vi "compare maps.vi"(10 "poolarimeter map path":path=path "test.tdms" caption="Filename", 11 "germanium map path":path=path "test.tdms" caption="Filename") -> (3 "germainium to polarimeter map":dbl[][](array[numeric]))   [LabVIEW 2018]
panel:
  out "map of germainium to polarimeter output along RF input unitary":T1(graph)
  out "Polarimeter Response Curve":cluster{dbl[], dbl[]}(graph)
  out "y offset 2":dbl
  out "y range 2":dbl
  out "x range 2":dbl
  out "x offset 2":dbl
  out "Germanium Response Curve":cluster{dbl[], dbl[]}(graph)
  out "y offset":dbl
  out "y range":dbl
  out "x range":dbl
  out "x offset":dbl
  out "Response Comparision":cluster{dbl[], dbl[]}[](graph)
  out "map of germainium to polarimeter output along RF input":T1(graph)
  out "germainium to polarimeter map unitary":dbl[][](array[numeric])
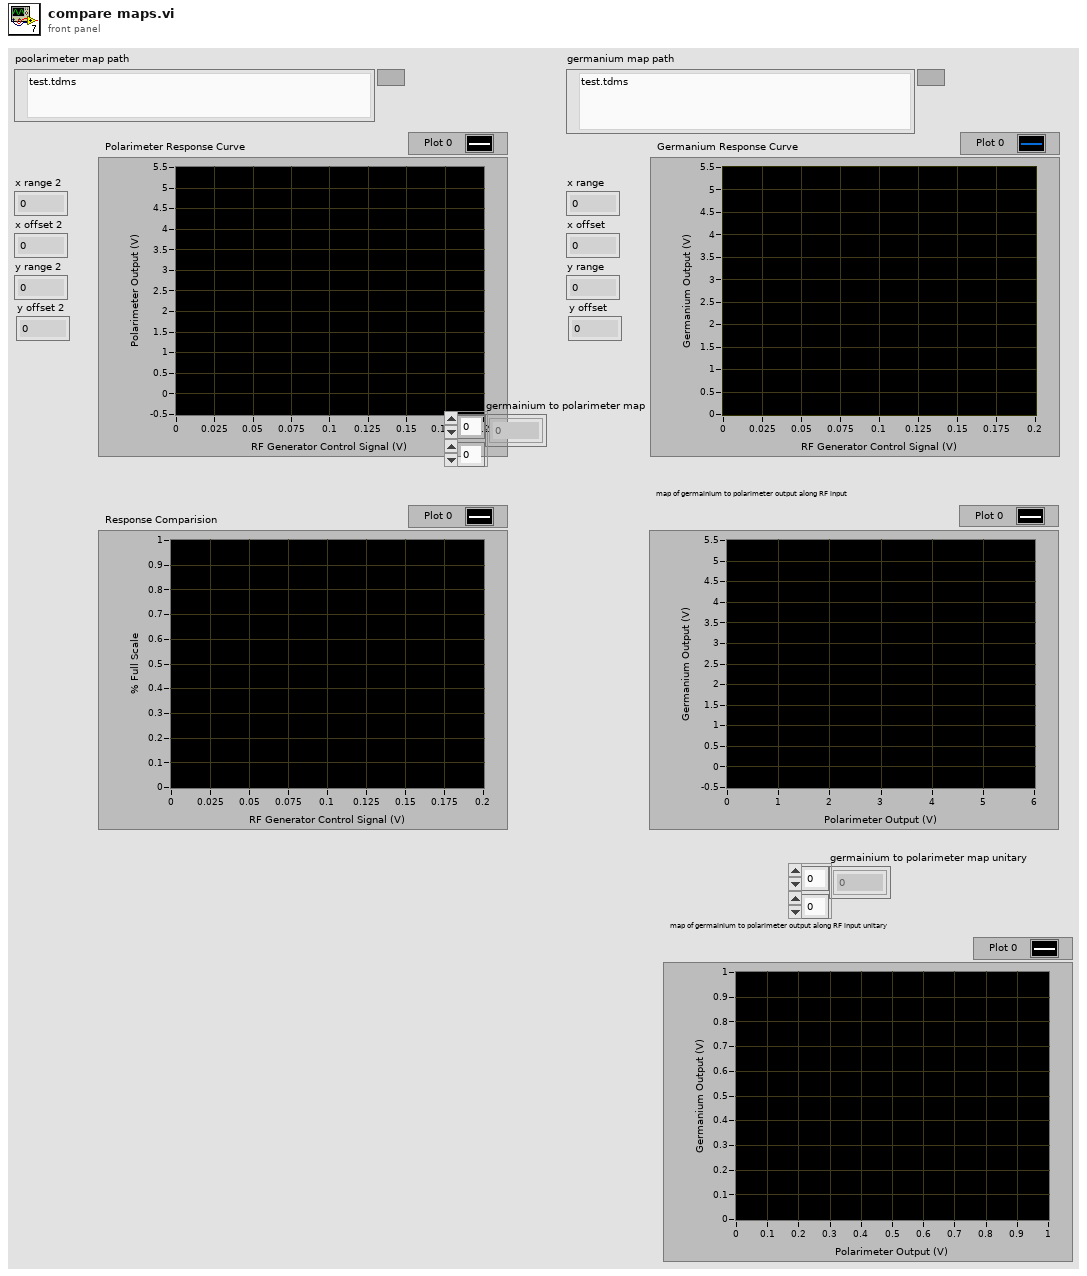
[diagram p1: front panel]
types:
  T1 = cluster{"Scaled Array":dbl[], "Scaled Array":dbl[]}
  T2 = cluster{"1N array":dbl[], "Scaled Array":dbl[]}[]
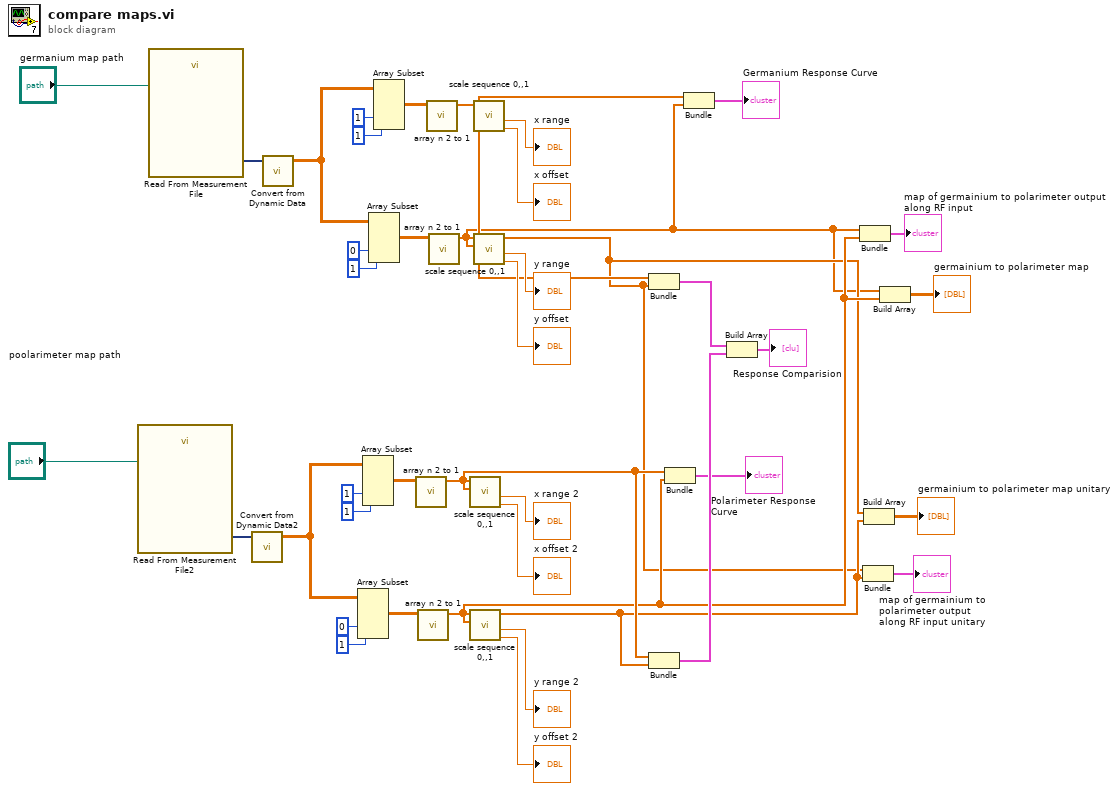
[diagram p0: block diagram]
diagram:
  n1 = call "Read From Measurement File2"("Filename"="poolarimeter map path") -> ("Signals"=w33:dynamicdata)  [unwired: 5 in, 5 out]
  n2 = call "Read From Measurement File"("Filename"="germanium map path") -> ("Signals"=w41:dynamicdata)  [unwired: 5 in, 5 out]
  n3 = call "Convert from Dynamic Data2"("Dynamic Data Type"=w33) -> ("Array"=w28:dbl[][])  [unwired: 3 in]
  n4 = call "Convert from Dynamic Data"("Dynamic Data Type"=w41) -> ("Array"=w36:dbl[][])  [unwired: 3 in]
  n5 = Array Subset(array=w28, index (col)=0 ("index"), length (col)=1 ("length")) -> (w26:dbl[][])  [unwired: 2 in]
  n6 = Array Subset(array=w28, index (col)=1 ("index"), length (col)=1 ("length")) -> (w27:dbl[][])  [unwired: 2 in]
  n7 = Array Subset(array=w36, index (col)=0 ("index"), length (col)=1 ("length")) -> (w34:dbl[][])  [unwired: 2 in]
  n8 = Array Subset(array=w36, index (col)=1 ("index"), length (col)=1 ("length")) -> (w35:dbl[][])  [unwired: 2 in]
  n9 = call "array n 2 to 1.vi"("2N array"=w27) -> ("1N array"=w8:dbl[])  [unwired: 10 in]
  n10 = call "array n 2 to 1.vi"("2N array"=w26) -> ("1N array"=w5:dbl[])  [unwired: 10 in]
  n11 = call "array n 2 to 1.vi"("2N array"=w35) -> ("1N array"=w10:dbl[])  [unwired: 10 in]
  n12 = call "array n 2 to 1.vi"("2N array"=w34) -> ("1N array"=w3:dbl[])  [unwired: 10 in]
  n13 = call "scale sequence 0,,1.vi"("Data"=w8, "map sequence"=w8) -> ("offset"=→"x offset 2":dbl, "range"=→"x range 2":dbl)  [unwired: 7 in, 1 out]
  n14 = call "scale sequence 0,,1.vi"("Data"=w5, "map sequence"=w5) -> ("offset"=→"y offset 2":dbl, "range"=→"y range 2":dbl, "Scaled Array"=w7:dbl[])  [unwired: 7 in]
  n15 = call "scale sequence 0,,1.vi"("Data"=w10, "map sequence"=w10) -> ("offset"=→"x offset":dbl, "range"=→"x range":dbl)  [unwired: 7 in, 1 out]
  n16 = call "scale sequence 0,,1.vi"("Data"=w3, "map sequence"=w3) -> ("offset"=→"y offset":dbl, "range"=→"y range":dbl, "Scaled Array"=w4:dbl[])  [unwired: 7 in]
  n17 = Bundle("1N array"=w10, "Scaled Array"=w4) -> (w22:cluster{"1N array":dbl[], "Scaled Array":dbl[]})  [unwired: 1 in]
  n18 = Bundle("1N array"=w8, "Scaled Array"=w7) -> (w16:cluster{"1N array":dbl[], "Scaled Array":dbl[]})  [unwired: 1 in]
  n19 = Bundle("1N array"=w8, "1N array"=w5) -> (→"Polarimeter Response Curve":cluster{"1N array":dbl[], "1N array":dbl[]})  [unwired: 1 in]
  n20 = Bundle("1N array"=w10, "1N array"=w3) -> (→"Germanium Response Curve":cluster{"1N array":dbl[], "1N array":dbl[]})  [unwired: 1 in]
  n21 = Build Array(w22, w16) -> (→"Response Comparision":T2)
  n22 = Bundle("1N array"=w3, "1N array"=w5) -> (→"map of germainium to polarimeter output along RF input":cluster{"1N array":dbl[], "1N array":dbl[]})  [unwired: 1 in]
  n23 = Bundle("Scaled Array"=w4, "Scaled Array"=w7) -> (→"map of germainium to polarimeter output along RF input unitary":T1)  [unwired: 1 in]
  n24 = Build Array(w4, w7) -> (→"germainium to polarimeter map unitary":dbl[][])
  n25 = Build Array(w3, w5) -> (→"germainium to polarimeter map":dbl[][])
